vi "main.eng.proc-start.vi"(8 "error in":errorcluster, 10 "params in":T1, 11 "Procs in":cluster{"Procedure":variant[]}[](array[cluster])) -> (0 "error out":errorcluster, 2 "isProcFound":bool, 3 "Procs out":cluster{"Procedure":variant[]}[](array[cluster]))   [LabVIEW 2024]
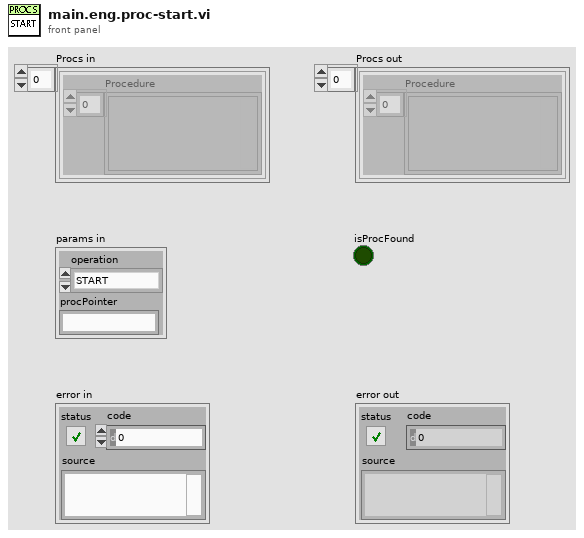
[diagram p1: front panel]
types:
  T1 = cluster{"operation":enum16{"START", "STOP"}, "procPointer":string}
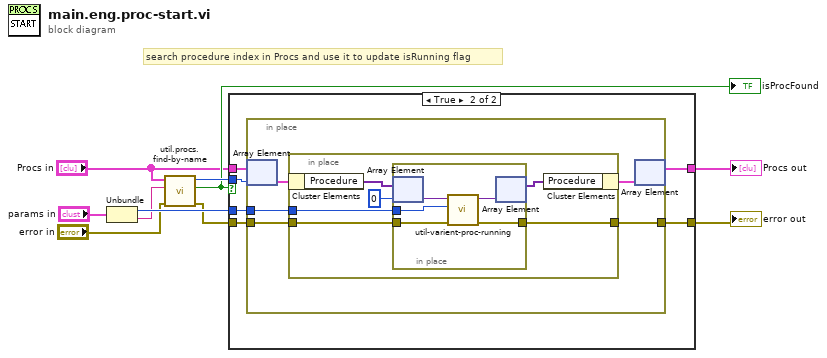
[diagram p0: block diagram]
diagram:
  # "search procedure index in Procs and use it to update isRunning flag"
  n1 = Unbundle("params in") -> ("operation"=w7:enum16{"START", "STOP"}, "procPointer"=w1:string)
  n2 = call "util.procs.find-by-name.vi"("error in"="error in", "ProcName in"=w1, "Procs in"="Procs in") -> ("error out"=w4:errorcluster, "Found?"=w6:bool, "procIndex"=w10:i32)  [unwired: 3 in, 3 out]
  "isProcFound" <- w6
  n3 = case shown="True" w6 {
    tunnel: w10 -> [_ w18]
    tunnel: [w12 w17] -> w9
    tunnel: "Procs in" -> [w12 w16]
    tunnel: w7 -> [_ w15]
    tunnel: [w11 w14] -> w5
    tunnel: w4 -> [w11 w13]
    frame False {
    }
    frame True {
      n4 = in-place {
        in-place-border: w15 -> [w21]
        in-place-border: [w20] -> w14
        in-place-border: w13 -> [w19]
        n5 = in-place-array #1(w16, w18) -> (w23:cluster{"Procedure":variant[]})
        n6 = in-place {
          in-place-border: w21 -> [w29]
          in-place-border: [w25] -> w20
          in-place-border: w19 -> [w24]
          n7 = in-place-cluster #2(w23) -> ("Procedure"=w28:variant[])
          n8 = in-place {
            in-place-border: w29 -> [w34]
            in-place-border: [w31] -> w25
            in-place-border: w24 -> [w30]
            n9 = in-place-array #3(w28, 0) -> (w33:variant)
            n10 = call "util-varient-proc-running.vi"("error in"=w30, "Enum"=w34, "Procedure in"=w33) -> ("error out"=w31:errorcluster, "Procedure out"=w32:variant)  [unwired: 7 in]
            n11 = in-place-array #3(w32) -> (w27:variant[])  [unwired: 1 out]
          }
          n12 = in-place-cluster #2("Procedure"=w27) -> (w22:cluster{"Procedure":variant[]})
        }
        n13 = in-place-array #1(w22) -> (w17:cluster{"Procedure":variant[]}[])  [unwired: 1 out]
      }
    }
  }
  "Procs out" <- w9
  "error out" <- w5
